vi "ExSubSetupADCQ.vi"(0 "Camera Handle":u32, 1 "Fast ADC":bool, 2 "ReadOut Port":u32 max=1 step=1, 3 "error in (no error)":errorcluster, 4 "ADC Gain":u32) -> (5 "Camera Handle":u32, 6 "ADC Speed (Khz)":u32, 7 "error out":errorcluster)   [LabVIEW 2010]
panel:
  # "Setup CoolSnap ADC\nThis sub VI sets the\nreadout port, Avlanche\ngain, ADC (fast or slow)\nand the gain for ADC.\nIt returns the ADC speed\nselected in Khz"
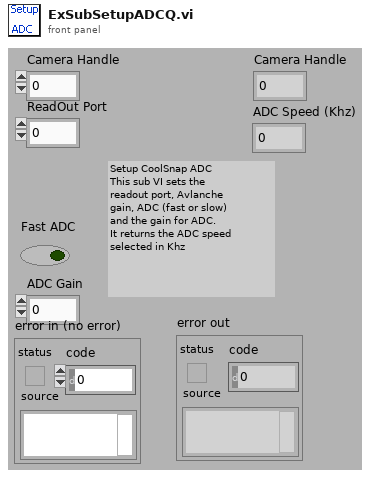
[diagram p1: front panel]
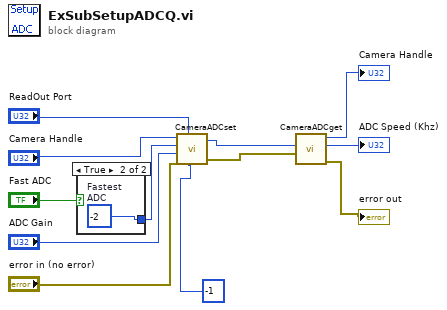
[diagram p0: block diagram]
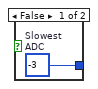
[diagram p2: hidden frame]
diagram:
  n1 = case shown="True" "Fast ADC" {
    tunnel: [w13 w14] -> w8
    frame False {
      w13 = -3  # Slowest ADC
    }
    frame True {
      w14 = -2  # Fastest ADC
    }
  }
  n2 = call <userlib>:"CameraADCset.vi"("ADC offset"=-1, "Read Out port"="ReadOut Port", "error in (no error)"="error in (no error)", "ADC Gain"="ADC Gain", "ADC Speed"=w8, "Camera Handle"="Camera Handle") -> ("error out"=w2:errorcluster, "Camera Handle"=w1:u32)
  n3 = call <userlib>:"CameraADCget.vi"("Camera handle"=w1, "error in (no error)"=w2) -> ("Camera handle"=→"Camera Handle":u32, "ADC Speed"=→"ADC Speed (Khz)":i32, "error out"=→"error out":errorcluster)  [unwired: 5 out]
